vi "from string.vi"(8 "error in":errorcluster, 9 "data":string, 10 "version":string, 11 "Polynomial Scale configuration in":refnum<class "Polynomial Scale configuration.lvclass">) -> (0 "error out":errorcluster, 3 "Polynomial Scale configuration out":refnum<class "Polynomial Scale configuration.lvclass">)   [LabVIEW 2013, in "Polynomial Scale configuration.lvclass"]
doc: "Provides an interface for loading a module configuration from a file or other serialized data source. It is recommended that all children of this class store data in two sets--data required for its own initialization, and any data required for parent initialization--and that each implementation uses the <b>Call Parent Method</b> primitive to de-serialize parent information. As a result, it is expected that every module configuration class calls <b>component configuration.lvclass:From String.vi</b>."
uses:
  Polynomial Scale configuration.lvclass
  <vilib>/NI/DCAF Modules/DCAF Scaling/module/configuration/Scaling configuration.lvclass
  Polynomial Scale configuration.lvclass/Polynomial Scale configuration.ctl
  <vilib>/NI/Tag Bus Module Framework/module configuration/TBM module configuration.lvclass
  <vilib>/NI/Configuration Framework/serializable configuration/NISE_CEF_serializable configuration.lvclass
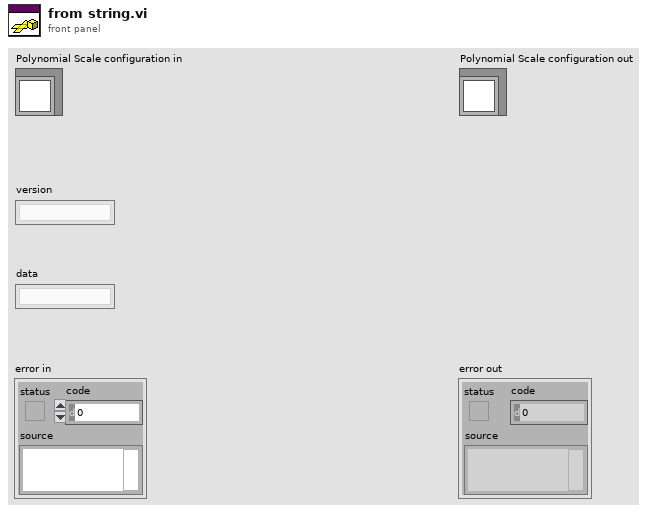
[diagram p1: front panel]
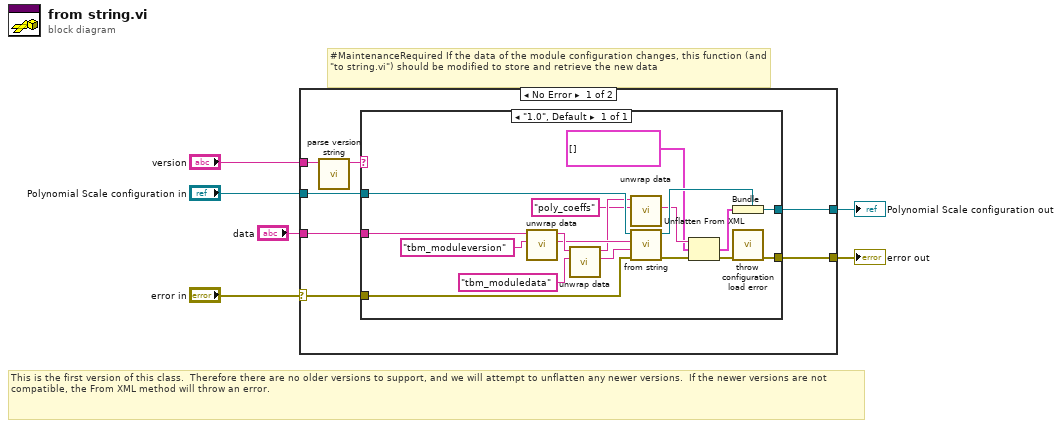
[diagram p0: block diagram]
diagram:
  # "#MaintenanceRequired If the data of the module configuration changes, this function (and \"to string.vi\") should be modified to store and retrieve the new data"
  # "This is the first version of this class.  Therefore there are no older versions to support, and we will attempt to unflatten any newer versions.  If the newer versions are not compatible, the From XML method will throw an error."
  n1 = case shown="No Error" "error in" {
    selector: "error in" -> [w7 w33]
    tunnel: "data" -> [w13 _]
    tunnel: "Polynomial Scale configuration in" -> [w12 w32]
    tunnel: [w11 w32] -> w5
    tunnel: [w10 w33] -> w4
    tunnel: "version" -> [w9 _]
    frame No Error {
      n2 = call <vilib>:"parse version string.vi"("full version"=w9) -> ("major.minor version"=w8:string)  [unwired: 7 in, 3 out]
      n3 = case shown="\"1.0\", Default" w8 {
        tunnel: w13 -> [w27]
        tunnel: w7 -> [w26]
        tunnel: w12 -> [w31]
        tunnel: [w21] -> w11
        tunnel: [w29] -> w10
        frame "1.0", Default {
          n4 = call <vilib>:"unwrap data.vi"("identifier"="tbm_moduleversion" ("additional identifier"), "data to unwrap"=w27) -> ("unwrapped data"=w22:string, "remaining string"=w28:string)  [unwired: 8 in]
          n5 = call <vilib>:"unwrap data.vi"("identifier"="tbm_moduledata" ("additional identifier"), "data to unwrap"=w28) -> ("unwrapped data"=w24:string, "remaining string"=w20:string)  [unwired: 8 in]
          n6 = call <vilib>:"unwrap data.vi"("identifier"="poly_coeffs" ("additional identifier"), "data to unwrap"=w20) -> ("unwrapped data"=w18:string)  [unwired: 8 in, 1 out]
          n7 = call-parent "from string.vi"("error in"=w26, "data"=w24, "version"=w22, "Scaling configuration in"=w31) -> ("error out"=w17:errorcluster, "Scaling configuration out"=w30:refnum<class "Polynomial Scale configuration.lvclass">)  [unwired: 6 in]
          n8 = Unflatten From XML(xml string=w18, type=cluster{"coeffs":dbl[]}[] [] ("coeff sets"), error in (no error)=w17) -> (value=w14:cluster{"coeffs":dbl[]}[], error out=w16:errorcluster)
          n9 = Bundle(cluster=w30, w14) -> (w21:refnum<class "Polynomial Scale configuration.lvclass">)
          n10 = call <vilib>:"throw configuration load error.vi"("error in"=w16) -> ("error out"=w29:errorcluster)  [unwired: 10 in]
        }
      }
    }
    frame Error {
    }
  }
  "error out" <- w4
  "Polynomial Scale configuration out" <- w5
